vi "delay.vi"(3 "Error In":errorcluster, 5 "time (ms)":u32) -> (0 "Error Out":errorcluster, 2 "resulting string":string)   [LabVIEW 2014]
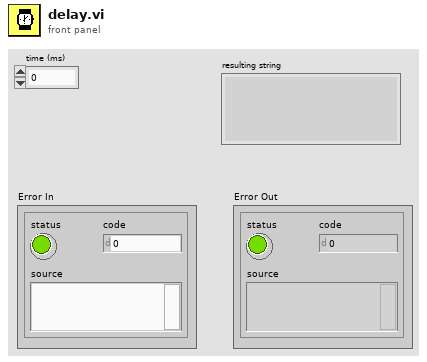
[diagram p1: front panel]
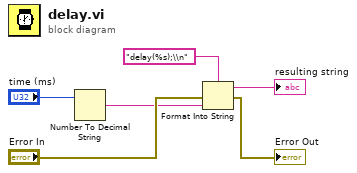
[diagram p0: block diagram]
diagram:
  n1 = Number To Decimal String(number="time (ms)") -> (decimal integer string=w4:string)  [unwired: 1 in]
  n2 = Format Into String(format string="delay(%s);\\n", error in="Error In", w4) -> (resulting string=→"resulting string":string, error out=→"Error Out":errorcluster)  [unwired: 1 in]
